vi "Carica da QUALIBUS.vi"(11 "Codice":string="192619") -> (3 "Dati caricati":string[][](array[string]))   [LabVIEW 2019]
uses:
  Globals.vi
  <vilib>/addons/database/Connection.llb/DB Tools Open Connec (String).vi
  <vilib>/addons/database/Connection.llb/Conn Execute.vi
  <vilib>/addons/database/Recordset.llb/Rec Destroy - Connection.vi
  <vilib>/addons/database/Recordset.llb/Rec Fetch Recordset Data (R).vi
  <vilib>/addons/database/_DB Variant To Data/Database Variant To Data.xnode
  <vilib>/addons/database/NI_Database_API.lvlib
panel:
  in  "connection information":path=path "C:/Lavori_in_corso_Tecnico4/C2018044_Oberti/Codice/Archivio/Nuovo documento di testo.udl"
  # "192585 - pompe eex\n192607 - pompa\n190007 - motore ca\n192454 - motore eex\n190524 - motore cc\n190003 - generico\n190002 - generatore\n192494 - trasformatore"
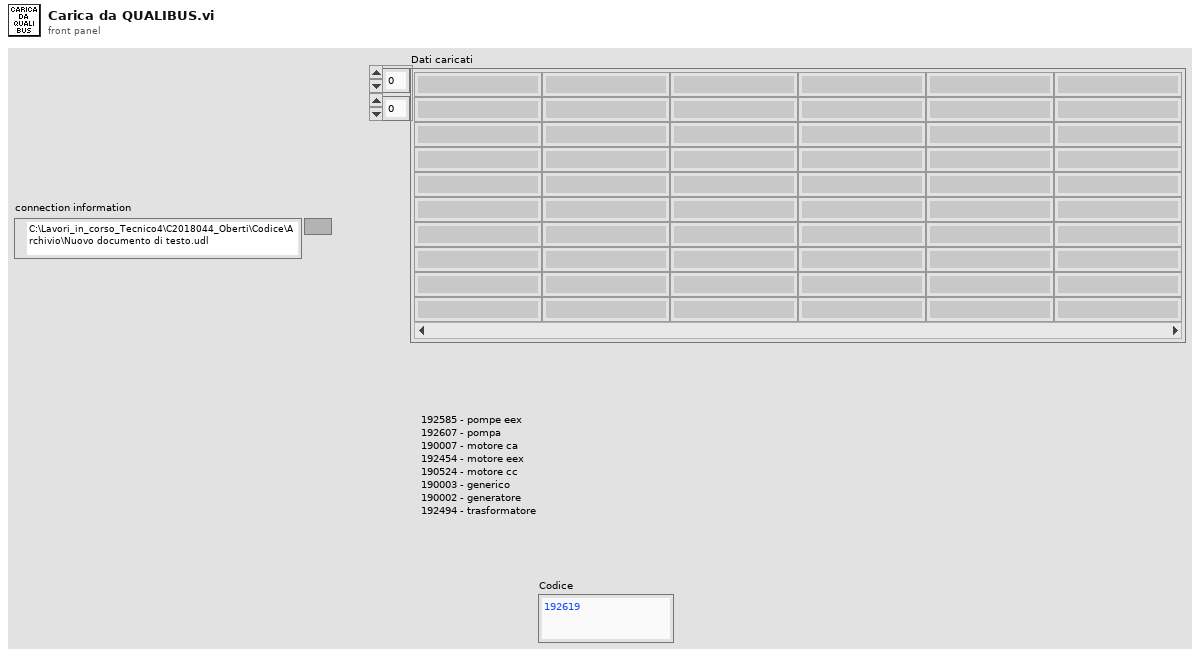
[diagram p1: front panel]
types:
  T1 = typedef "NI_Database_API.lvlib/Conn ObjectReference.ctl" = refnum<k1>
  T2 = typedef "NI_Database_API.lvlib/Rec ObjectReference.ctl" = refnum<k1>
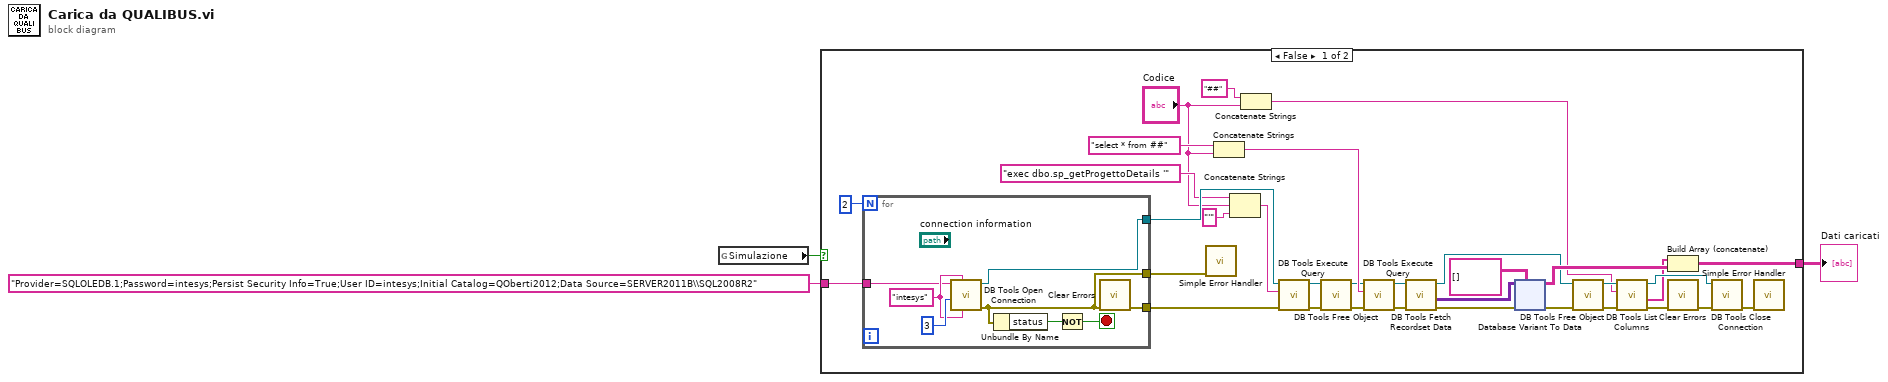
[diagram p0: block diagram]
diagram:
  n1 = global read "Globals.vi" "Simulazione"() -> (w1:bool)
  n2 = case shown="False" w1 {
    tunnel: [w32 _] -> w3
    tunnel: "Provider=SQLOLEDB.1;Password=intesys;Persist Security Info=True;User ID=intesys;Initial Catalog=QOberti2012;Data Source=SERVER2011B\\SQL2008R2" ("userID") -> [w4 _]
    frame False {
      n3 = for {
        N: 2 -> [_]
        tunnel: [w39] -> w6
        tunnel: [w42] -> w33
        tunnel: [w38] -> w5
        tunnel: w4 -> [w37]
        stop <- w40 stop-if-true
        w43 = "intesys" ("userID")
        n4 = call-poly <vilib>:"DB Tools Open Connection.vi"("password"=w43, "userID"=w43, "connection timeout (15)"=3, "connection information"=w37) -> ("error out"=w38:errorcluster, "connection reference"=w42:T1)  [unwired: 4 in]
        n5 = Unbundle By Name(w38) -> ("status"=w41:bool)
        n6 = Not(x=w41) -> (.not. x?=w40:bool)
        n7 = call <vilib>:"Clear Errors.vi"("error in (no error)"=w38) -> ("error out"=w39:errorcluster)  [unwired: 5 in, 1 out]
      }
      n8 = call <vilib>:"Simple Error Handler.vi"("error in (no error)"=w5) -> ()  [unwired: 4 in, 5 out]
      n9 = Concatenate Strings("select * from ##" ("SQL query"), "Codice") -> (w19:string)
      n10 = Concatenate Strings("exec dbo.sp_getProgettoDetails '" ("SQL query"), "Codice", "'" ("string")) -> (w21:string)
      n11 = Concatenate Strings("##" ("string"), "Codice") -> (w17:string)
      n12 = call-poly <vilib>:"DB Tools Execute Query.vi"("error in (no error)"=w6, "SQL query"=w21, "connection reference"=w33) -> ("error out"=w13:errorcluster, "recordset reference"=w15:T2)  [unwired: 5 in]
      n13 = call-poly <vilib>:"DB Tools Free Object.vi"("error in (no error)"=w13, "recordset reference"=w15) -> ("error out"=w12:errorcluster, "connection reference"=w14:T1)  [unwired: 8 in]
      n14 = call-poly <vilib>:"DB Tools Execute Query.vi"("error in (no error)"=w12, "SQL query"=w19, "connection reference"=w14) -> ("error out"=w24:errorcluster, "recordset reference"=w28:T2)  [unwired: 5 in]
      n15 = call-poly <vilib>:"DB Tools Fetch Recordset Data.vi"("error in (no error)"=w24, "recordset reference"=w28) -> ("error out"=w11:errorcluster, "recordset data"=w31:variant[][], "recordset reference out"=w27:T2)  [unwired: 3 in]
      n16 = xnode "Database Variant To Data"("database variant"=w31, "error in (no error)"=w11, "type"=string[][] []) -> ("data"=w29:string[][], "error out"=w10:errorcluster)
      n17 = call-poly <vilib>:"DB Tools Free Object.vi"("error in (no error)"=w10, "recordset reference"=w27) -> ("error out"=w16:errorcluster, "connection reference"=w26:T1)  [unwired: 8 in]
      n18 = call <vilib>:"DB Tools List Columns.vi"("error in (no error)"=w16, "table"=w17, "connection reference"=w26) -> ("error out"=w9:errorcluster, "columns"=w25:string[], "connection reference out"=w34:T1)  [unwired: 1 in, 1 out]
      n19 = Build Array (concatenate)(w25, w29) -> (w32:string[][])
      n20 = call <vilib>:"Clear Errors.vi"("error in (no error)"=w9) -> ("error out"=w35:errorcluster)  [unwired: 5 in, 1 out]
      n21 = call <vilib>:"DB Tools Close Connection.vi"("error in (no error)"=w35, "connection reference"=w34) -> ("error out"=w36:errorcluster)  [unwired: 5 in]
      n22 = call <vilib>:"Simple Error Handler.vi"("error in (no error)"=w36) -> ()  [unwired: 4 in, 5 out]
    }
    frame True {
    }
  }
  "Dati caricati" <- w3
